vi "Request_int_JSON.vi"(0 "reference in":T1, 5 "method":string, 7 "params":refnum<class "JSON Null.lvclass">, 9 "id":i32, 11 "error in (no error)":errorcluster) -> (4 "reference out":T1, 6 "response":refnum<class "JSON Null.lvclass">, 15 "error out":errorcluster)   [LabVIEW 2017, in "JSON_RPC_client.lvlib"]
uses:
  JSON_RPC_client.lvlib
  reference.ctl
  <vilib>/httpClient/ClientHandle.ctl
  <vilib>/NI/JSON Support for LabVIEW/JSON Data Classes/JSON Datatype/JSON Null.lvclass
  <vilib>/NI/JSON Support for LabVIEW/JSON Data Classes/JSON Object/New JSON Object (Empty).vi
  <vilib>/NI/JSON Support for LabVIEW/JSON Data Classes/JSON Object/Insert Key Value Pair.vi
  <vilib>/NI/JSON Support for LabVIEW/JSON Data Classes/JSON Object/Insert Key Value Pair (Single String).vi
  <vilib>/NI/JSON Support for LabVIEW/JSON Data Classes/JSON Object/Insert Key Value Pair (Single).vi
  <vilib>/NI/JSON Support for LabVIEW/JSON Data Classes/JSON Object/Insert Key Value Pair (Single Numeric).vi
  <vilib>/httpClient/POSTBuffer.vi
  <vilib>/NI/JSON Support for LabVIEW/JSON Data Classes/JSON Helper/Parsing/Parse Value.vi
  <vilib>/NI/JSON Support for LabVIEW/JSON Data Classes/JSON Object/Set Object Parameters XNode/Set Object Parameters.xnode
  <vilib>/NI/JSON Support for LabVIEW/JSON Data Classes/JSON Object/JSON Object.lvclass
  <vilib>/httpClient/LabVIEWHTTPClient.lvlib
  <vilib>/NI/JSON Support for LabVIEW/JSON Data Classes/JSON Helper/JSON Helper.lvclass
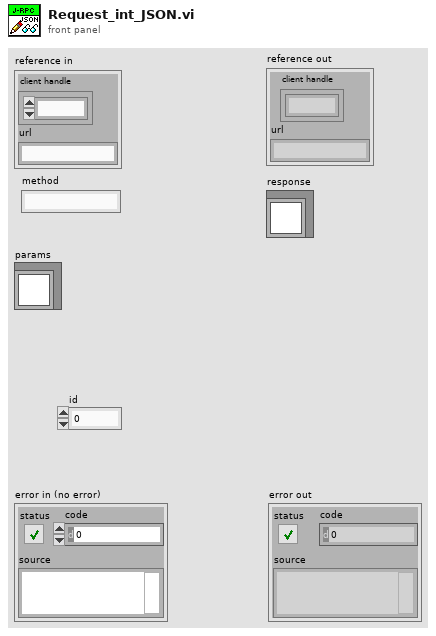
[diagram p1: front panel]
types:
  T1 = typedef "JSON_RPC_client.lvlib/reference.ctl" = cluster{"client handle":T2, "url":string}
  T2 = typedef "LabVIEWHTTPClient.lvlib/ClientHandle.ctl" = refnum<k1>
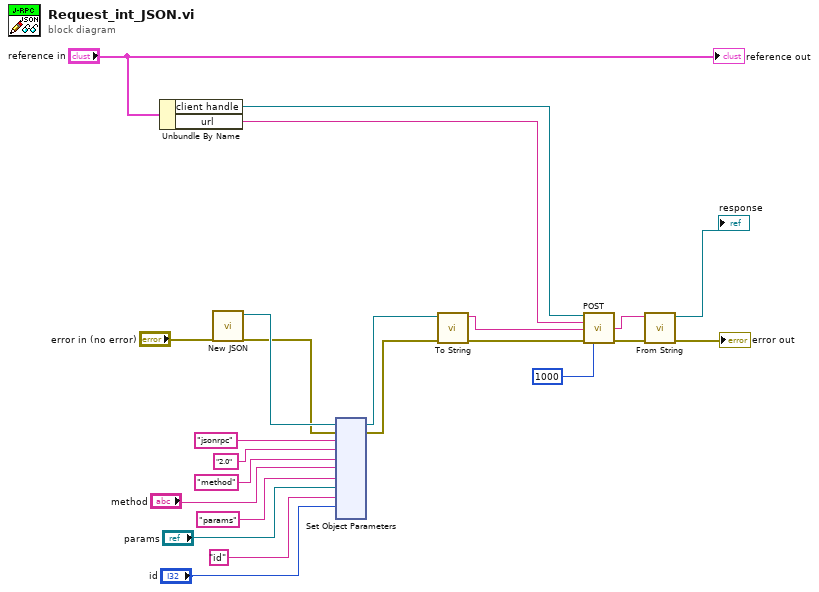
[diagram p0: block diagram]
diagram:
  n1 = Unbundle By Name("reference in") -> ("client handle"=w22:T2, "url"=w21:string)
  n2 = call-poly <vilib>:"New JSON.vi"("error in (no error)"="error in (no error)") -> ("error out"=w10:errorcluster, "JSON Object out"=w16:refnum<class "JSON Object.lvclass">)  [unwired: 9 in]
  n3 = xnode "Set Object Parameters"("key"="jsonrpc" ("Name"), "key"="method" ("Name"), "key"="params" ("Name"), "key"="id" ("Name"), "parameter"="2.0" ("String"), "parameter"="method", "parameter"="params", "parameter"="id", "JSON Object In"=w16, "error in"=w10) -> ("JSON Object Out"=w9:refnum<class "JSON Object.lvclass">, "error out"=w8:errorcluster)  [unwired: 4 out]
  n4 = call-dynamic "To String.vi"("error in (no error)"=w8, "JSON Object in"=w9) -> ("error out"=w2:errorcluster, "String"=w3:string)  [unwired: 8 in]
  n5 = call-poly <vilib>:"POST.vi"("client handle"=w22, "url"=w21, "buffer"=w3, "error in (no error)"=w2, "timeout (10000)"=1000) -> ("body"=w19:string, "error out"=w20:errorcluster)  [unwired: 7 in, 2 out]
  n6 = call <vilib>:"From String.vi"("error in (no error)"=w20, "JSON String"=w19) -> ("error out"=→"error out":errorcluster, "JSON out"=→"response":refnum<class "JSON Null.lvclass">)  [unwired: 8 in]
  "reference out" <- "reference in"
